vi "Import DPIDs.vi"(8 "error in (no error)":errorcluster, 11 "Node Ptr":u64 format="%.0x") -> (0 "error out":errorcluster)   [LabVIEW 2019, in "Diagnostics Addon System Explorer.lvlib"]
uses:
  Diagnostics Addon System Explorer.lvlib
  <vilib>/NI VeriStand/Custom Device API/Custom Device API.lvlib
  <vilib>/NI VeriStand/Custom Device Tools/Custom Device Utility Library/Custom Device Utility Library.lvlib
  Shared/Types/DPID.Rate.ctl
  Shared/Diagnostics Addon Shared.lvlib
  Shared/Types/DPID.ctl
  Types/DPID.Export.ctl
panel:
  in  "Tag":string
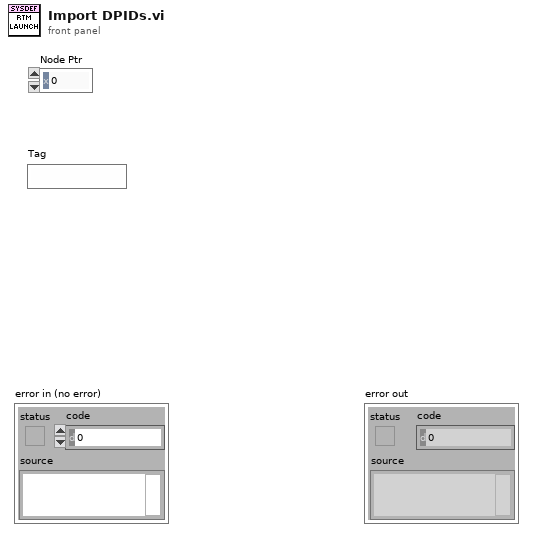
[diagram p1: front panel]
types:
  T1 = typedef "Diagnostics Addon Shared.lvlib/DPID.ctl" = cluster{"DPID ID":u8, "Speed":T2, "PIDs":u16[]}
  T2 = typedef "Diagnostics Addon Shared.lvlib/DPID.Rate.ctl" = enum16{"Slow", "Medium", "Fast"}
  T3 = typedef "Diagnostics Addon System Explorer.lvlib/DPID.Export.ctl" = cluster{"Name":string, "Description":string, "DPID":T1}
  T4 = typedef "Diagnostics Addon System Explorer.lvlib/Frame.Export.ctl" = cluster{"Name":string, "Description":string, "ID":u32, "Signals":T5[]}
  T5 = typedef "Diagnostics Addon Shared.lvlib/Signal.ctl" = cluster{"Start Bit":u32, "Length":u32, "Scaling Factor":dbl, "Scaling Offset":dbl, "Minimum":dbl, "Maximum":dbl, "Data Type":u32, "Byte Order":u32, "Default Value":dbl, "Name":string, "Units":string, "Description":string}
  T6 = typedef "Custom Device API.lvlib/Custom Device Item Ref.ctl" = u64
  T7 = typedef "Custom Device API.lvlib/Custom Device Item Info.ctl" = cluster{"Name":string, "Is Channel":bool, "GUID":string, "Is Waveform":bool}
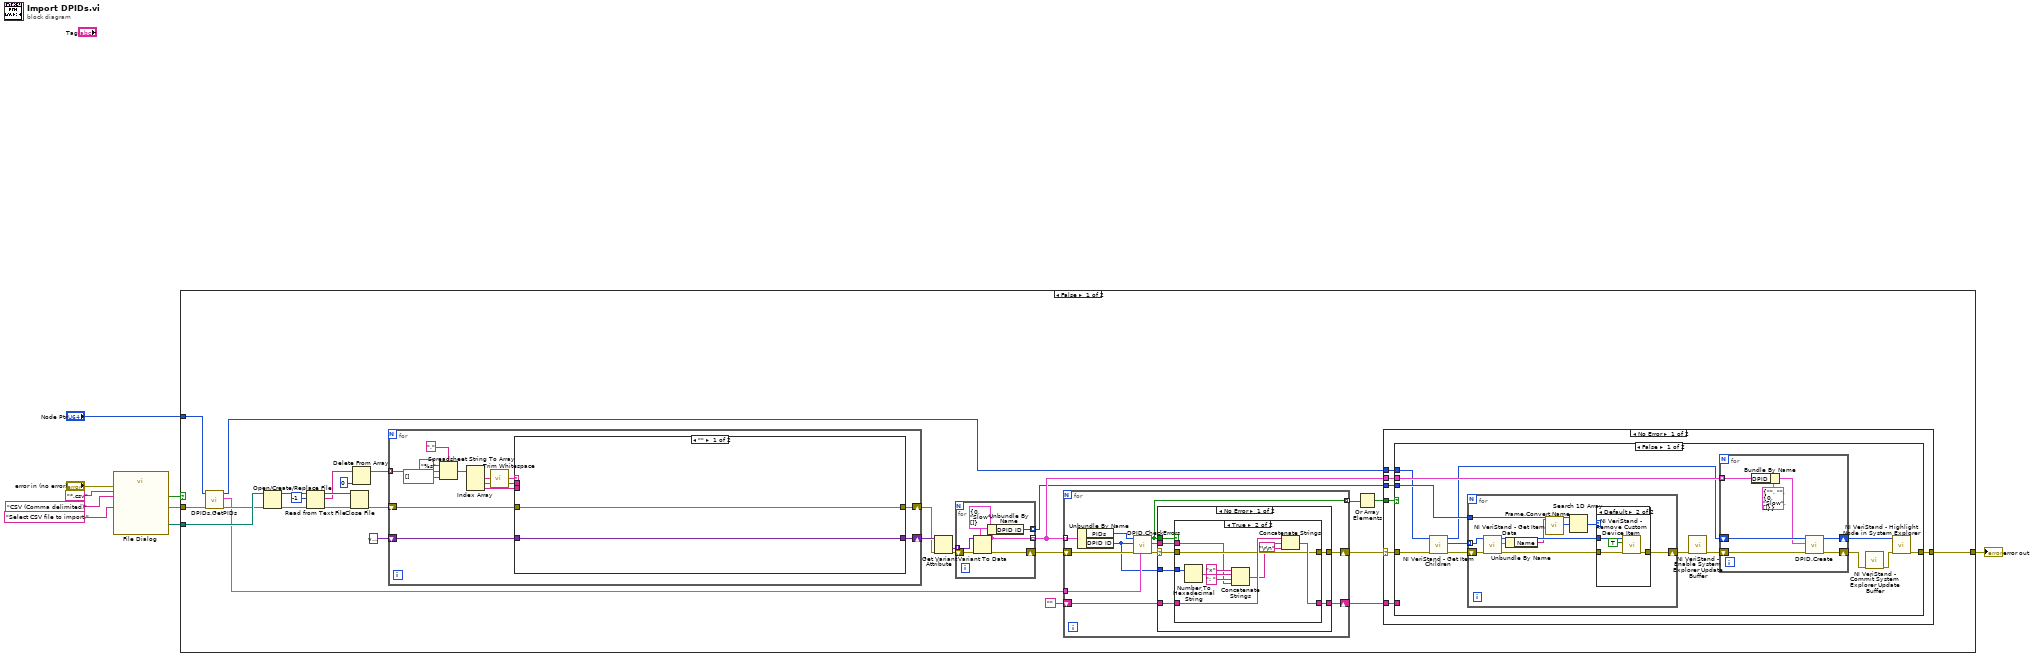
[diagram p0: block diagram]
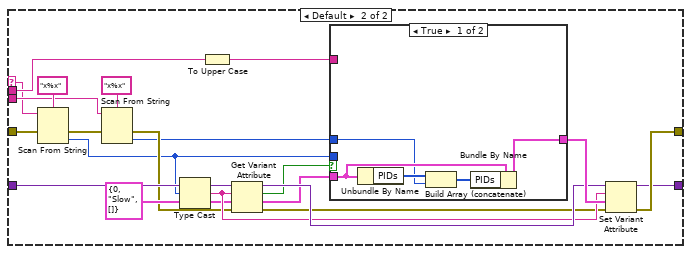
[diagram p2: hidden frame]
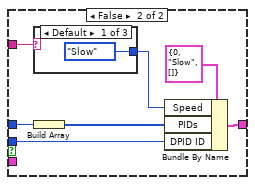
[diagram p3: hidden frame]
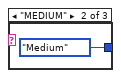
[diagram p4: hidden frame]
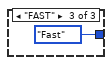
[diagram p5: hidden frame]
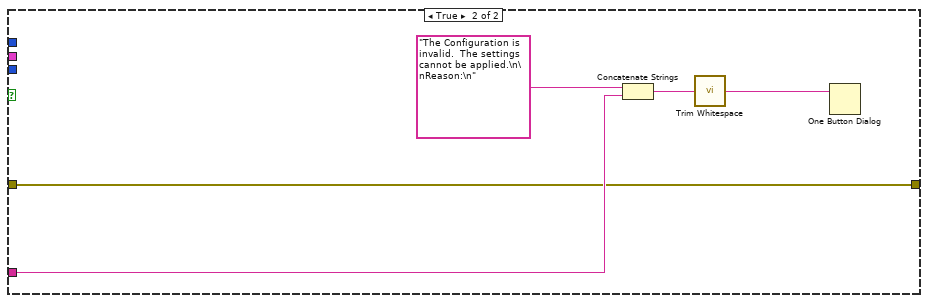
[diagram p7: hidden frame]
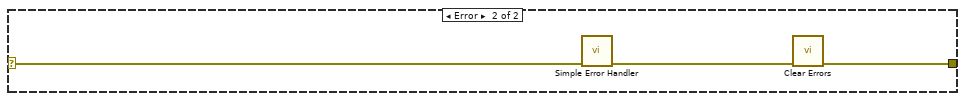
[diagram p8: hidden frame]
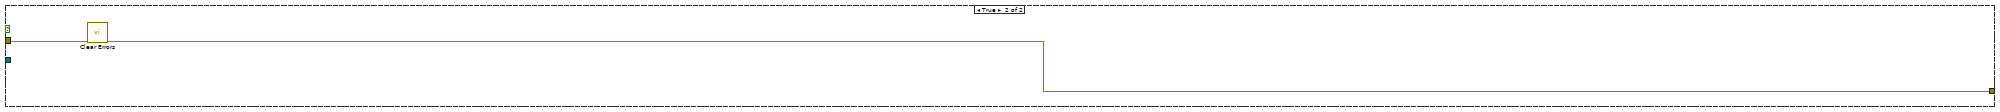
[diagram p11: hidden frame]
diagram:
  n1 = call "File Dialog"("prompt"="Select CSV file to import.", "error in"="error in (no error)", "pattern (all files)"="*.csv" ("pattern label"), "pattern label"="CSV (Comma delimited)") -> ("selected path"=w4:path, "cancelled"=w6:bool, "error out"=w5:errorcluster)  [unwired: 8 in, 1 out]
  n2 = case shown="False" w6 {
    tunnel: w5 -> [w14 w179]
    tunnel: w4 -> [w34 _]
    tunnel: "Node Ptr" -> [w12 _]
    tunnel: [w18 w178] -> w2
    frame False {
      n3 = call "DPIDs.GetPIDs.vi"("error in (no error)"=w14, "Item Ref in"=w12) -> ("error out"=w13:errorcluster, "PIDs"=w10:T4[], "Section Ref out"=w11:T6)  [unwired: 7 in]
      n4 = Open/Create/Replace File(file path (use dialog)=w34, error in=w13) -> (refnum out=w37:refnum<file>, error out=w38:errorcluster)  [unwired: 4 in, 1 out]
      n5 = Read from Text File(file (use dialog)=w37, count=-1, error in=w38) -> (refnum out=w36:refnum<file>, text=w26:string[], error out=w35:errorcluster)  [unwired: 1 in, 1 out]
      n6 = Close File(refnum=w36, error in=w35) -> (error out=w32:errorcluster)  [unwired: 1 out]
      n7 = Delete From Array(array=w26, index=0) -> (array with subset deleted=w25:string[])  [unwired: 1 in, 1 out]
      n8 = for {
        tunnel: w25 -> [w47] mode=indexing
        shift-right: [w49] -> w29
        shift-left: w32 -> [w50]
        shift-right: [w48] -> w30
        shift-left: variant -> [w51]
        n9 = Spreadsheet String To Array(delimiter (Tab)=",", format string="%s", spreadsheet string=w47, array type (2D Dbl)=string[] []) -> (array=w43:string[])
        n10 = Index Array(array=w43) -> (element #1=w40:string, element #2=w41:string, element #3=w42:string)  [unwired: 3 in]
        n11 = call <vilib>:"Trim Whitespace.vi"("string"=w40) -> ("trimmed string"=w39:string)  [unwired: 1 in]
        n12 = case shown="\"\"" w39 {
          selector: w39 -> [_ w54]
          tunnel: w51 -> [w53 w73]
          tunnel: w50 -> [w52 w72]
          tunnel: [w52 w69] -> w49
          tunnel: [w53 w68] -> w48
          tunnel: w42 -> [_ w58]
          tunnel: w41 -> [_ w57]
          frame "" {
          }
          frame Default {
            n13 = Scan From String(format string="x%x", input string=w54, error in=w72) -> (error out=w60:errorcluster, output 1=w55:u32)  [unwired: 2 in, 2 out]
            n14 = Scan From String(format string="x%x", input string=w58, error in=w60) -> (error out=w59:errorcluster, output 1=w56:u32)  [unwired: 2 in, 2 out]
            n15 = Type Cast(x=w55) -> (*(type *) &x=w67:string)  [unwired: 1 in]
            n16 = To Upper Case(1:w57) -> (0:w62:string)
            n17 = Get Variant Attribute(Variant=w73, name=w67, default value (empty Variant)=T1 {"DPID ID"=0, "Speed"=enum."Slow", "PIDs"=[]} ("DPID"), error in=w59) -> (duplicate Variant=w70:variant, found=w66:bool, value=w65:T1, error out=w63:errorcluster)
            n18 = case shown="True" w66 {
              tunnel: w55 -> [_ w80]
              tunnel: w62 -> [_ w82]
              tunnel: [w76 w86] -> w71
              tunnel: w65 -> [w79 _]
              tunnel: w56 -> [w75 w84]
              frame True {
                n19 = Unbundle By Name(w79) -> ("PIDs"=w78:u16[])
                n20 = Build Array (concatenate)(w78, w75) -> (w77:u32[])
                n21 = Bundle By Name(cluster=w79, "PIDs"=w77) -> (w76:T1)
              }
              frame False {
                n22 = case shown="Default" w82 {
                  tunnel: [DPID.Rate."Slow" ("Speed") DPID.Rate."Medium" ("Speed") DPID.Rate."Fast" ("Speed")] -> w81
                  frame Default {
                  }
                  frame "MEDIUM" {
                  }
                  frame "FAST" {
                  }
                }
                n23 = Build Array(w84) -> (w83:u32[])
                n24 = Bundle By Name(cluster=T1 {"DPID ID"=0, "Speed"=enum."Slow", "PIDs"=[]} ("DPID"), "Speed"=w81, "PIDs"=w83, "DPID ID"=w80) -> (w86:T1)
              }
            }
            n25 = Set Variant Attribute(Variant=w70, name=w67, value=w71, error in=w63) -> (Variant out=w68:variant, error out=w69:errorcluster)  [unwired: 1 out]
          }
        }
      }
      n26 = Get Variant Attribute(Variant=w30, error in=w29) -> (values=w28:variant[], error out=w27:errorcluster)  [unwired: 2 in, 2 out]
      n27 = for {
        tunnel: w28 -> [w95] mode=indexing
        shift-right: [w93] -> w17
        shift-left: w27 -> [w94]
        tunnel: [w92] -> w19 mode=indexing
        tunnel: [w91] -> w16 mode=indexing
        n28 = Variant To Data(error in=w94, type=T1 {"DPID ID"=0, "Speed"=enum."Slow", "PIDs"=[]} ("DPID"), Variant=w95) -> (data=w92:T1, error out=w93:errorcluster)
        n29 = Unbundle By Name(w92) -> ("DPID ID"=w91:u8)
      }
      n30 = for {
        tunnel: w19 -> [w156] mode=indexing
        shift-right: [w153] -> w15
        shift-left: w17 -> [w152]
        shift-right: [w155] -> w20
        shift-left: "" -> [w154]
        tunnel: [w149] -> w22 mode=indexing
        tunnel: w10 -> [w148]
        n31 = Unbundle By Name(w156) -> ("PIDs"=w147:u16[], "DPID ID"=w146:u8)
        n32 = call "DPID.CheckErrors.vi"("Existing PIDs"=w148, "error in (no error)"=w152, "DPID ID"=w146, "PIDs"=w147) -> ("error out"=w151:errorcluster, "Reason"=w150:string, "Error?"=w149:bool)  [unwired: 5 in]
        n33 = case shown="No Error" w151 {
          selector: w151 -> [w159 w176]
          tunnel: w149 -> [w162 _]
          tunnel: w150 -> [w163 _]
          tunnel: [w161 w177] -> w155
          tunnel: w154 -> [w160 w177]
          tunnel: [w158 w176] -> w153
          tunnel: w146 -> [w157 _]
          frame No Error {
            n34 = case shown="True" w162 {
              tunnel: w163 -> [_ w167]
              tunnel: [w165 w175] -> w161
              tunnel: w160 -> [w165 w174]
              tunnel: w159 -> [w164 w172]
              tunnel: [w164 w172] -> w158
              tunnel: w157 -> [_ w169]
              frame False {
              }
              frame True {
                n35 = Number To Hexadecimal String(2:w169) -> (0:w171:string)  [unwired: 1 in]
                n36 = Concatenate Strings("x" ("string"), w171, ": " ("string"), w167) -> (w166:string)
                n37 = Concatenate Strings(w174, w166, "\r\n") -> (w175:string)
              }
            }
          }
          frame Error {
          }
        }
      }
      n38 = Or Array Elements(Boolean array=w22) -> (logical OR=w21:bool)
      n39 = case shown="No Error" w15 {
        selector: w15 -> [w98 w145]
        tunnel: w21 -> [w102 _]
        tunnel: w20 -> [w101 _]
        tunnel: w19 -> [w100 _]
        tunnel: [w99 w143] -> w18
        tunnel: w11 -> [w97 _]
        tunnel: w16 -> [w96 _]
        frame No Error {
          n40 = case shown="False" w102 {
            tunnel: w101 -> [_ w140]
            tunnel: w98 -> [w106 w139]
            tunnel: w100 -> [w111 _]
            tunnel: [w110 w139] -> w99
            tunnel: w97 -> [w105 _]
            tunnel: w96 -> [w107 _]
            frame False {
              n41 = call <vilib>:"NI VeriStand - Get Item Children.vi"("error in (no error)"=w106, "Item Ref in"=w105) -> ("error out"=w109:errorcluster, "Child Refs"=w108:T6[], "Item Ref out"=w103:T6)  [unwired: 6 in, 1 out]
              n42 = for {
                shift-right: [w120] -> w104
                shift-left: w109 -> [w124]
                tunnel: w108 -> [w123] mode=indexing
                tunnel: w107 -> [w122]
                n43 = call <vilib>:"NI VeriStand - Get Item Data.vi"("error in (no error)"=w124, "Item Ref in"=w123) -> ("error out"=w121:errorcluster, "Item Info"=w125:T7, "Item Ref out"=w119:T6)  [unwired: 7 out]
                n44 = Unbundle By Name(w125) -> ("Name"=w117:string)
                n45 = call "Frame.Convert.Name.vi"("VS Frame Name"=w117) -> ("ID"=w116:u16)  [unwired: 9 in, 1 out]
                n46 = Search 1D Array(1D array=w122, element=w116) -> (index of element=w118:i32)  [unwired: 1 in]
                n47 = case shown="Default" w118 {
                  tunnel: w121 -> [w126 w130]
                  tunnel: [w126 w129] -> w120
                  tunnel: w119 -> [_ w128]
                  frame -1 {
                  }
                  frame Default {
                    n48 = call <vilib>:"NI VeriStand - Remove Custom Device Item.vi"("error in (no error)"=w130, "Force Delete (F)"=TRUE, "Item Ref in"=w128) -> ("error out"=w129:errorcluster)  [unwired: 7 in, 1 out]
                  }
                }
              }
              n49 = call <vilib>:"NI VeriStand - Enable System Explorer Update Buffer.vi"("error in (no error)"=w104) -> ("error out"=w114:errorcluster)  [unwired: 10 in]
              n50 = for {
                shift-right: [w136] -> w113
                shift-left: w114 -> [w137]
                shift-right: [w134] -> w115
                shift-left: w103 -> [w135]
                tunnel: w111 -> [w132] mode=indexing
                n51 = Bundle By Name(cluster=T3 {"Name"="", "Description"="", "DPID"={"DPID ID"=0, "Speed"=enum."Slow", "PIDs"=[]}} ("DPID"), "DPID"=w132) -> (w131:T3)
                n52 = call "DPID.Create.vi"("error in (no error)"=w137, "DPID"=w131, "Section Ptr"=w135) -> ("error out"=w136:errorcluster, "Parent Ref out"=w134:T6)  [unwired: 7 in]
              }
              n53 = call <vilib>:"NI VeriStand - Commit System Explorer Update Buffer.vi"("error in (no error)"=w113) -> ("error out"=w112:errorcluster)  [unwired: 10 in]
              n54 = call <vilib>:"NI VeriStand - Highlight Node in System Explorer.vi"("error in (no error)"=w112, "Item Ref in"=w115) -> ("error out"=w110:errorcluster)  [unwired: 8 in, 1 out]
            }
            frame True {
              n55 = Concatenate Strings("The Configuration is invalid.  The settings cannot be applied.\n\nReason:\n" ("message"), w140) -> (w142:string)
              n56 = call <vilib>:"Trim Whitespace.vi"("string"=w142) -> ("trimmed string"=w138:string)  [unwired: 1 in]
              n57 = One Button Dialog(message=w138) -> ()  [unwired: 1 in, 1 out]
            }
          }
        }
        frame Error {
          n58 = call <vilib>:"Simple Error Handler.vi"("error in (no error)"=w145) -> ("error out"=w144:errorcluster)  [unwired: 4 in, 4 out]
          n59 = call <vilib>:"Clear Errors.vi"("error in (no error)"=w144) -> ("error out"=w143:errorcluster)  [unwired: 5 in, 1 out]
        }
      }
    }
    frame True {
      n60 = call <vilib>:"Clear Errors.vi"("error in (no error)"=w179) -> ("error out"=w178:errorcluster)  [unwired: 5 in, 1 out]
    }
  }
  "error out" <- w2
